vi "Calculate Hold-In Measurements.vi"(0 "Stage Waveform Section":dbl[](array[numeric])) -> (4 "Max Stage":dbl, 6 "Min Stage":dbl, 8 "Avg Stage":dbl, 10 "Avg Max Stage":dbl, 15 "Avg Min Stage":dbl)   [LabVIEW 2015, in "Fuel Injector Analysis Addon Engine.lvlib"]
uses:
  Fuel Injector Analysis Addon Engine.lvlib
  <vilib>/Analysis/baseanly.llb/Mean (DBL).vi
  <vilib>/Analysis/NI_AALBase.lvlib
  <vilib>/Analysis/NI_AAL_SigProc.lvlib
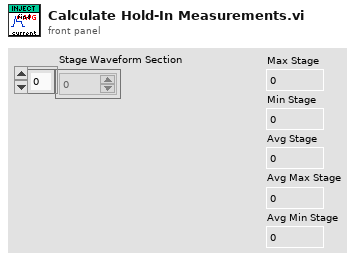
[diagram p1: front panel]
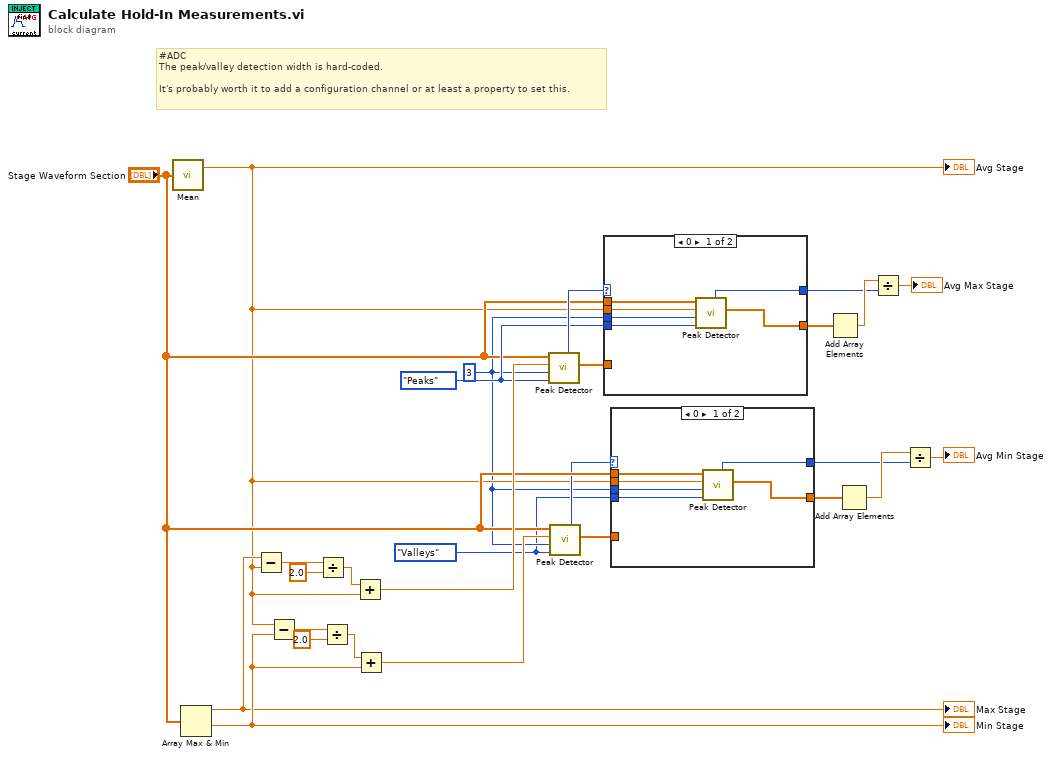
[diagram p0: block diagram]
diagram:
  w4 = 3 ("width")
  w3 = enum32{"Peaks", "Valleys"}."Valleys" ("peaks/valleys")
  w9 = enum32{"Peaks", "Valleys"}."Peaks" ("peaks/valleys")
  # "#ADC \nThe peak/valley detection width is hard-coded.\n\nIt's probably worth it to add a configuration channel or at least a property to set this."
  n1 = call-poly <vilib>:"Mean.vi"("X"="Stage Waveform Section") -> ("mean"=w5:dbl)  [unwired: 1 out]
  "Avg Stage" <- w5
  n2 = Array Max & Min(array="Stage Waveform Section") -> (max value=w18:dbl, min value=w21:dbl)  [unwired: 2 out]
  "Max Stage" <- w18
  "Min Stage" <- w21
  n3 = Subtract(x=w18, y=w5) -> (x-y=w15:dbl)
  n4 = Subtract(x=w5, y=w21) -> (x-y=w23:dbl)
  n5 = Divide(x=w15, y=2.0) -> (x/y=w17:dbl)
  n6 = Divide(x=w23, y=2.0) -> (x/y=w20:dbl)
  n7 = Add(x=w17, y=w5) -> (x+y=w14:dbl)
  n8 = Add(x=w20, y=w21) -> (x+y=w19:dbl)
  n9 = call <vilib>:"Peak Detector.vi"("peaks/valleys"=w9, "width"=w4, "threshold"=w14, "X"="Stage Waveform Section") -> ("Amplitudes"=w11:dbl[], "# found"=w13:i32)  [unwired: 3 in, 3 out]
  n10 = call <vilib>:"Peak Detector.vi"("peaks/valleys"=w3, "width"=w4, "threshold"=w19, "X"="Stage Waveform Section") -> ("Amplitudes"=w8:dbl[], "# found"=w6:i32)  [unwired: 3 in, 3 out]
  n11 = case shown="0" w13 {
    selector: w13 -> [_ w34]
    tunnel: "Stage Waveform Section" -> [w33 _]
    tunnel: [w32 w35] -> w12
    tunnel: w11 -> [_ w35]
    tunnel: [w31 w34] -> w10
    tunnel: w4 -> [w30 _]
    tunnel: w9 -> [w29 _]
    tunnel: w5 -> [w28 _]
    frame 0 {
      n12 = call <vilib>:"Peak Detector.vi"("peaks/valleys"=w29, "width"=w30, "threshold"=w28, "X"=w33) -> ("Amplitudes"=w32:dbl[], "# found"=w31:i32)  [unwired: 3 in, 3 out]
    }
    frame Default {
    }
  }
  n13 = case shown="0" w6 {
    selector: w6 -> [_ w42]
    tunnel: "Stage Waveform Section" -> [w41 _]
    tunnel: [w40 w43] -> w2
    tunnel: w8 -> [_ w43]
    tunnel: [w39 w42] -> w1
    tunnel: w4 -> [w38 _]
    tunnel: w3 -> [w37 _]
    tunnel: w5 -> [w36 _]
    frame 0 {
      n14 = call <vilib>:"Peak Detector.vi"("peaks/valleys"=w37, "width"=w38, "threshold"=w36, "X"=w41) -> ("Amplitudes"=w40:dbl[], "# found"=w39:i32)  [unwired: 3 in, 3 out]
    }
    frame Default {
    }
  }
  n15 = Add Array Elements(numeric array=w12) -> (sum=w24:dbl)
  n16 = Add Array Elements(numeric array=w2) -> (sum=w25:dbl)
  n17 = Divide(x=w24, y=w10) -> (x/y=→"Avg Max Stage":dbl)
  n18 = Divide(x=w25, y=w1) -> (x/y=→"Avg Min Stage":dbl)
